vi "write_randoms.vi"() -> ()   [LabVIEW 2018]
panel:
  in  "file path (use dialog)":path
  in  "stop":bool
  out "String":string
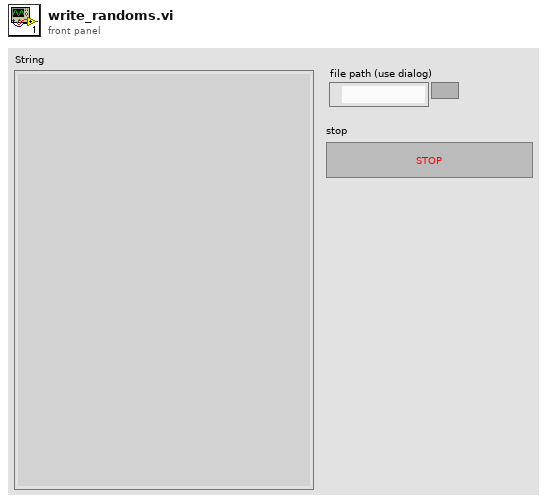
[diagram p1: front panel]
types:
  T1 = enum16{"open", "replace", "create", "open or create", "replace or create", "replace or create with confirmation"}
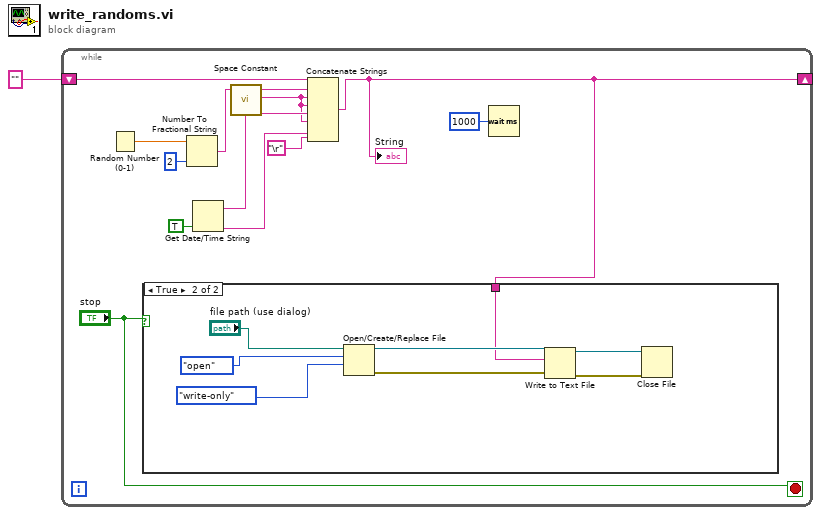
[diagram p0: block diagram]
diagram:
  n1 = while {
    shift-right: [w3] -> _
    shift-left: "" -> [w13]
    stop <- "stop" stop-if-true
    n2 = Random Number (0-1)() -> (number: 0 to 1=w12:dbl)
    n3 = Number To Fractional String(number=w12, precision (6)=i16 2) -> (F-format string=w10:string)  [unwired: 2 in]
    n4 = Get Date/Time String(want seconds? (F)=TRUE) -> (date string=w8:string, time string=w6:string)  [unwired: 2 in]
    n5 = call <vilib>:"Space Constant.vi"() -> ("String"=w7:string)
    n6 = Concatenate Strings(w13, w10, w7, w7, w8, w7, w6, "\r") -> (w3:string)
    "String" <- w3
    n7 = case shown="True" "stop" {
      tunnel: w3 -> [_ w16]
      frame False {
      }
      frame True {
        n8 = Open/Create/Replace File(file path (use dialog)="file path (use dialog)", operation (0:open)=T1."open", access (0:read/write)=enum16{"read/write", "read-only", "write-only"}."write-only") -> (refnum out=w18:refnum<file>, error out=w17:errorcluster)  [unwired: 3 in, 1 out]
        n9 = Write to Text File(file (use dialog)=w18, text=w16, error in=w17) -> (refnum out=w15:refnum<file>, error out=w14:errorcluster)  [unwired: 1 in, 1 out]
        n10 = Close File(refnum=w15, error in=w14) -> ()  [unwired: 2 out]
      }
    }
    n11 = Wait (ms)(milliseconds to wait=u32 1000) -> ()  [unwired: 1 out]
  }
